vi "GetAutotoolRegionsRuntime.vi"(0 "XRef":T16, 1 "State In":T7) -> (14 "Regions":T2, 15 "Fatal Error Out":T1)   [LabVIEW 2020, in "FlexBlock.xnode"]
uses:
  FlexBlock.xnode
  <vilib>/XNodeSupport/XNodeXNodeRef.ctl
  State.ctl
  <vilib>/XNodeSupport/XNodeAutotoolRegions.ctl
  <vilib>/XNodeSupport/XNodeAutotoolRegion.ctl
  <vilib>/XNodeSupport/XNodeRect32.ctl
  <vilib>/XNodeSupport/XNodeInt.ctl
  <vilib>/XNodeSupport/XNodeTools.ctl
  <vilib>/XNodeSupport/XNodeErrorCluster.ctl
  <vilib>/XNodeSupport/NI_XNodeSupport.lvlib
  FlexBlocks/Terminal Direction.ctl
  FlexBlocks/FlexBlocks.lvlib
  FlexBlocks/Value Mode.ctl
  FlexBlocks/Terminal State.ctl
  FlexBlocks/Type Descriptor.ctl
  FlexBlocks/Errors.ctl
  <vilib>/picture/picture.llb/imagedata.ctl
  FlexBlocks/Special Terminal.ctl
  FlexBlocks/Calculated Sizes.ctl
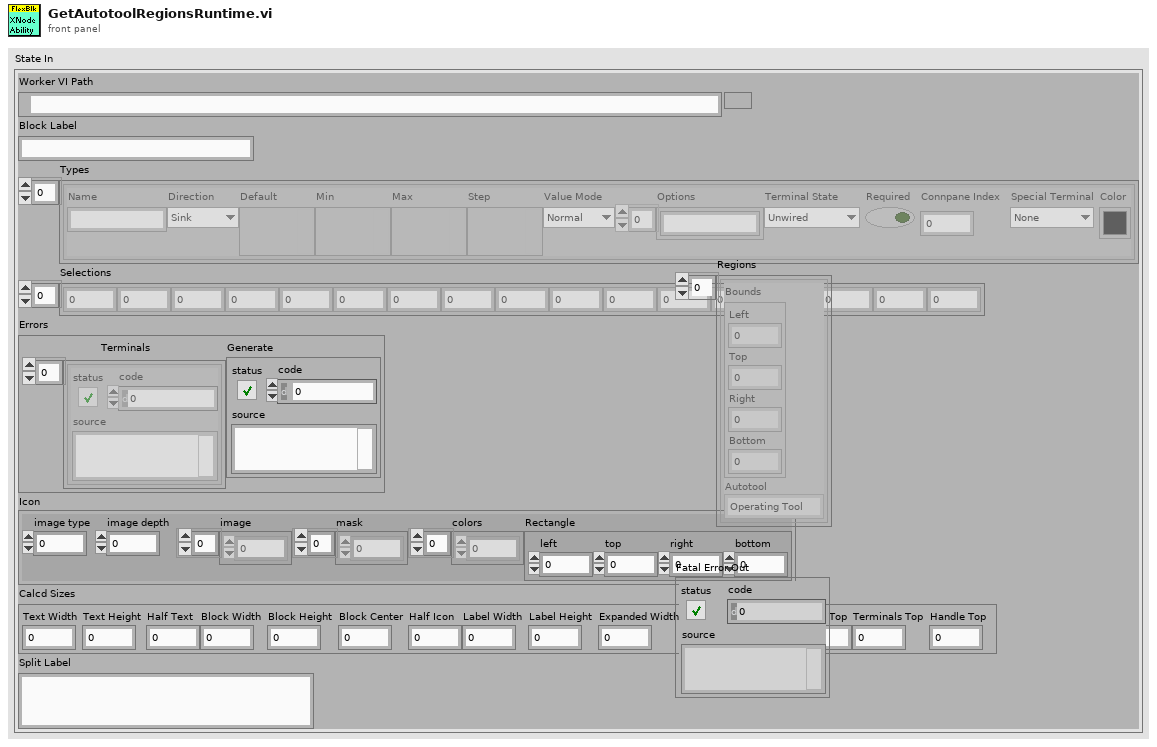
[diagram p1: front panel]
types:
  T1 = typedef "NI_XNodeSupport.lvlib/XNodeErrorCluster.ctl" = errorcluster
  T2 = typedef "NI_XNodeSupport.lvlib/XNodeAutotoolRegions.ctl" = T3[]
  T3 = typedef "NI_XNodeSupport.lvlib/XNodeAutotoolRegion.ctl" = cluster{"Bounds":T4, "Autotool":T6}
  T4 = typedef "NI_XNodeSupport.lvlib/XNodeRect32.ctl" = cluster{"Left":T5, "Top":T5, "Right":T5, "Bottom":T5}
  T5 = typedef "NI_XNodeSupport.lvlib/XNodeInt.ctl" = i32
  T6 = typedef "NI_XNodeSupport.lvlib/XNodeTools.ctl" = enum32{"Operating Tool", "Placement Tool", "Labelling Tool", "Wiring Tool", "Scroll Tool", "Breakpoint Tool", "Probe Tool", "Auto Tool"}
  T7 = typedef "FlexBlock.xnode/State.ctl" = cluster{"Worker VI Path":path, "Block Label":string, "Types":T8[], "Selections":i32[], "Errors":T13, "Icon":T14, "Calcd Sizes":T15, "Split Label":string}
  T8 = typedef "FlexBlocks.lvlib/Type Descriptor.ctl" = cluster{"Name":string, "Direction":T9, "Default":variant, "Min":variant, "Max":variant, "Step":variant, "Value Mode":T10, "Options":string[], "Terminal State":T11, "Required":bool, "Connpane Index":i32, "Special Terminal":T12, "Color":u32}
  T9 = typedef "FlexBlocks.lvlib/Terminal Direction.ctl" = enum16{"Sink", "Source"}
  T10 = typedef "FlexBlocks.lvlib/Value Mode.ctl" = enum16{"Normal", "Range", "Select"}
  T11 = typedef "FlexBlocks.lvlib/Terminal State.ctl" = enum16{"Unwired", "BadType", "BadRef", "Channel", "Value", "Control Ref"}
  T12 = typedef "FlexBlocks.lvlib/Special Terminal.ctl" = enum16{"None", "Action", "Init", "Tag", "State in", "State out", "Error"}
  T13 = typedef "FlexBlocks.lvlib/Errors.ctl" = cluster{"Terminals":errorcluster[], "Generate":errorcluster}
  T14 = typedef "imagedata.ctl" = cluster{"image type":i32, "image depth":i32, "image":u8[], "mask":u8[], "colors":u32[], "Rectangle":cluster{"left":i16, "top":i16, "right":i16, "bottom":i16}}
  T15 = typedef "FlexBlocks.lvlib/Calculated Sizes.ctl" = cluster{"Text Width":i32, "Text Height":i32, "Half Text":i32, "Block Width":i32, "Block Height":i32, "Block Center":i32, "Half Icon":i32, "Label Width":i32, "Label Height":i32, "Expanded Width":i32, "Half Label":i32, "Icon Top":i32, "Label Top":i32, "Terminals Top":i32, "Handle Top":i32}
  T16 = typedef "NI_XNodeSupport.lvlib/XNodeXNodeRef.ctl" = refnum<vi>
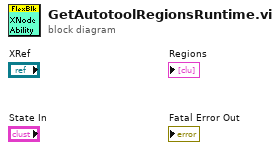
[diagram p0: block diagram]
diagram:
